vi "StandAloneTransient_Dynamic_Keithley2230_PSU_Configuration_V1.vi"(0 "VISA resource name":refnum<visa-resource-name>, 1 "POWER STATUS IN":bool, 5 "Input Array (Voltage,Current_Limit)":dbl[][](array[numeric]), 7 "Combination Scheme":u16(ring) items=["OFF", "SERIES", "PARALLEL"], 9 "Which Channels to Parallelize":u16(ring) items=["I1+I2", "ALL", "I2+I3"], 11 "error in":errorcluster) -> (3 "POWER STATUS OUT":bool, 4 "Array 4":dbl[][](array[numeric]), 6 "Array":string[](array[string]), 8 "read buffer":string, 15 "error out":errorcluster)   [LabVIEW 2019]
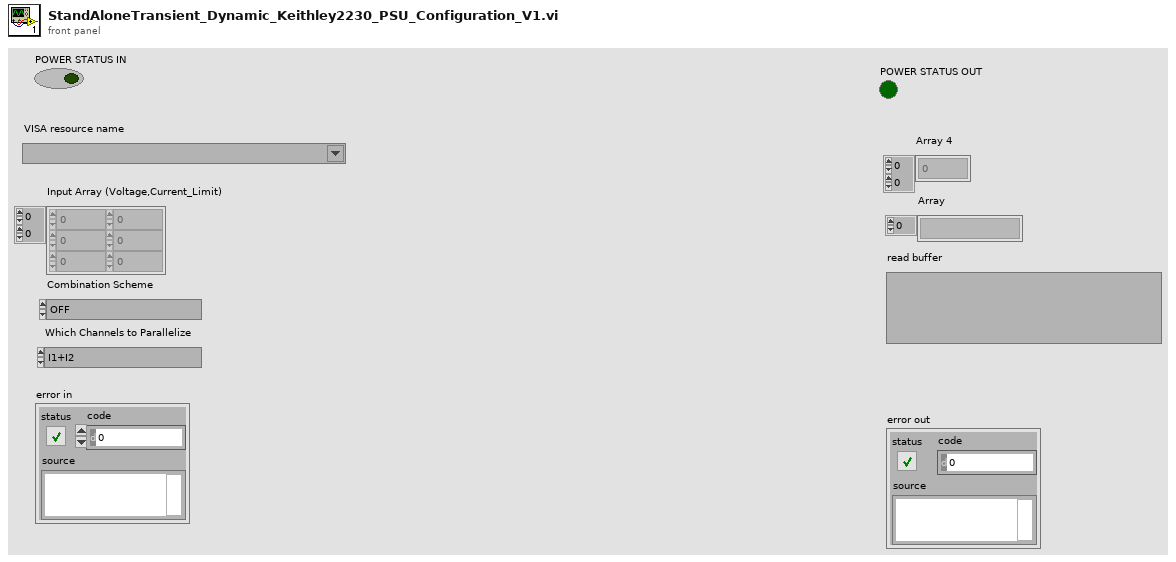
[diagram p1: front panel]
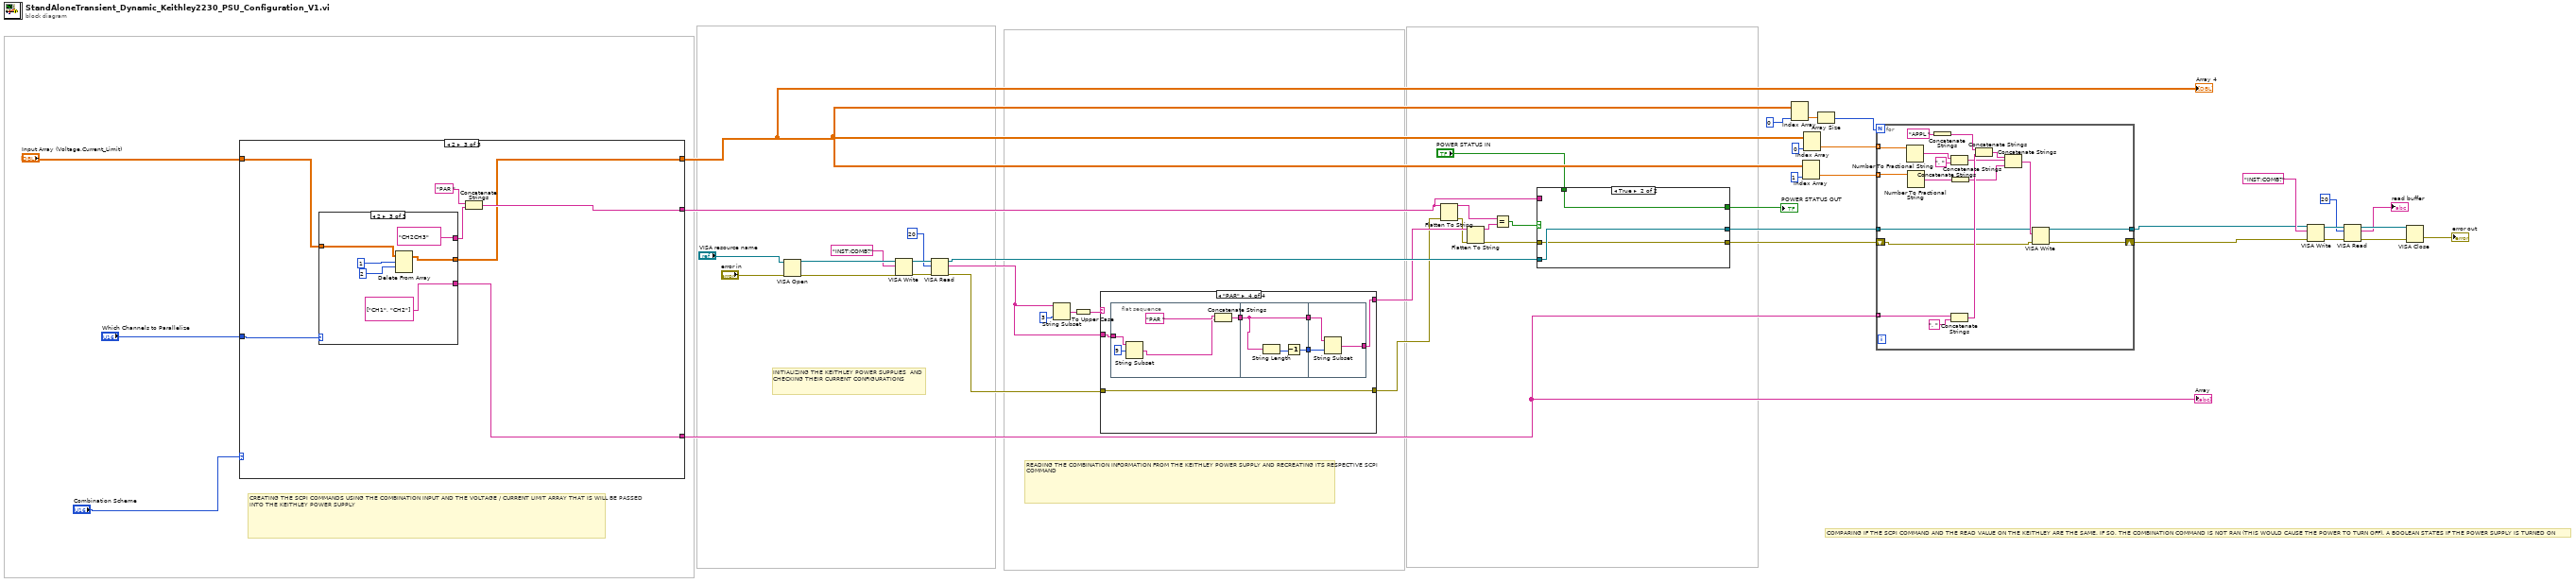
[diagram p0: block diagram]
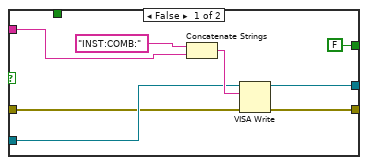
[diagram p2: hidden frame]
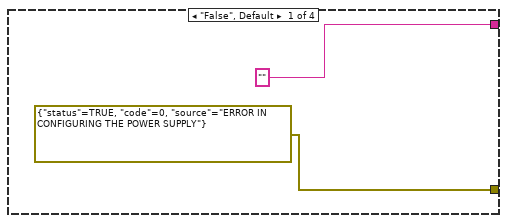
[diagram p3: hidden frame]
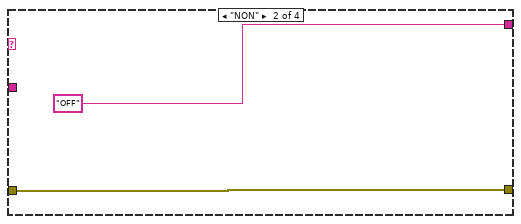
[diagram p4: hidden frame]
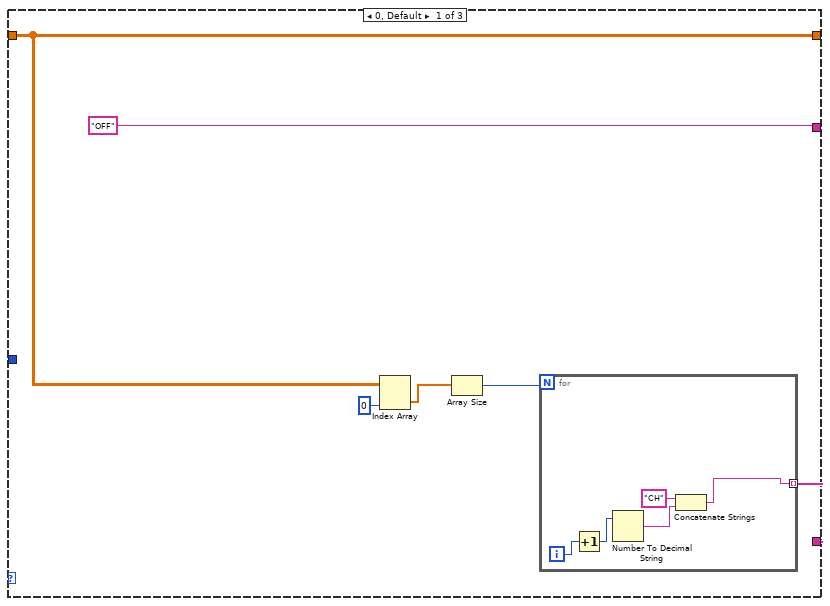
[diagram p6: hidden frame]
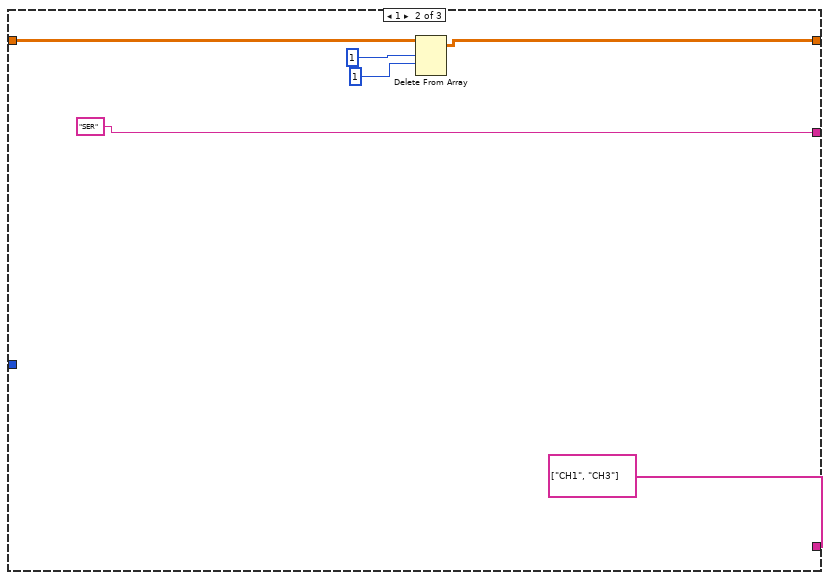
[diagram p7: hidden frame]
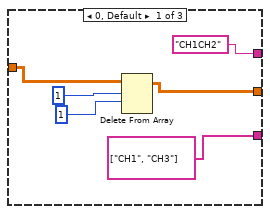
[diagram p8: hidden frame]
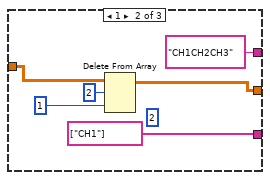
[diagram p9: hidden frame]
diagram:
  # "COMPARING IF THE SCPI COMMAND AND THE READ VALUE ON THE KEITHLEY ARE THE SAME. IF SO, THE COMBINATION COMMAND IS NOT RAN (THIS WOULD CAUSE THE POWER TO TURN OFF). A BOOLEAN STATES IF THE POWER SUPPLY IS TURNED ON"
  # "READING THE COMBINATION INFORMATION FROM THE KEITHLEY POWER SUPPLY AND RECREATING ITS RESPECTIVE SCPI COMMAND"
  # "CREATING THE SCPI COMMANDS USING THE COMBINATION INPUT AND THE VOLTAGE / CURRENT LIMIT ARRAY THAT IS WILL BE PASSED INTO THE KEITHLEY POWER SUPPLY"
  # "INITIALIZING THE KEITHLEY POWER SUPPLIES  AND CHECKING THEIR CURRENT CONFIGURATIONS"
  n1 = case shown="2" "Combination Scheme" {
    tunnel: ["OFF" "SER" w69] -> w16
    tunnel: "Which Channels to Parallelize" -> [_ _ w72]
    tunnel: "Input Array (Voltage,Current_Limit)" -> [w53 w63 w67]
    tunnel: [w53 w60 w66] -> w34
    tunnel: [w49 string[] ["CH1", "CH3"] w68] -> w35
    frame 0, Default {
      n2 = Index Array(array=w53, index (col)=0 ("disabled index (col)")) -> (element=w52:dbl[])  [unwired: 1 in]
      n3 = Array Size(array=w52) -> (size(s)=w50:i32)
      n4 = for {
        N: w50 -> [_]
        tunnel: [w55] -> w49 mode=indexing
        i -> [w58]
        n5 = Increment(x=w58) -> (x+1=w59:i32)
        n6 = Number To Decimal String(number=w59) -> (decimal integer string=w57:string)  [unwired: 1 in]
        n7 = Concatenate Strings("CH" ("string"), w57) -> (w55:string)
      }
    }
    frame 1 {
      n8 = Delete From Array(array=w63, length=1, index (row)=1) -> (array with subset deleted=w60:dbl[][])  [unwired: 1 in, 1 out]
    }
    frame 2 {
      n9 = case shown="2" w72 {
        tunnel: ["CH1CH2" "CH1CH2CH3" "CH2CH3"] -> w70
        tunnel: [string[] ["CH1", "CH3"] string[] ["CH1"] string[] ["CH1", "CH2"]] -> w68
        tunnel: w67 -> [w74 w82 w86]
        tunnel: [w73 w79 w87] -> w66
        frame 0, Default {
          n10 = Delete From Array(array=w74, length=1, index (row)=1) -> (array with subset deleted=w73:dbl[][])  [unwired: 1 in, 1 out]
        }
        frame 1 {
          (unwired) 2 ("index (row)")
          n11 = Delete From Array(array=w82, length=2, index (row)=1) -> (array with subset deleted=w79:dbl[][])  [unwired: 1 in, 1 out]
        }
        frame 2 {
          n12 = Delete From Array(array=w86, length=1, index (row)=2) -> (array with subset deleted=w87:dbl[][])  [unwired: 1 in, 1 out]
        }
      }
      n13 = Concatenate Strings("PAR ", w70) -> (w69:string)
    }
  }
  "Array 4" <- w34
  "Array" <- w35
  n14 = VISA Open(error in (no error)="error in", VISA resource name="VISA resource name") -> (VISA resource name=w31:refnum<visa-resource-name>, error out=w30:errorcluster)  [unwired: 3 in]
  n15 = VISA Write(VISA resource name=w31, write buffer="INST:COMB?", error in (no error)=w30) -> (VISA resource name out=w29:refnum<visa-resource-name>, error out=w28:errorcluster)  [unwired: 1 out]
  n16 = VISA Read(VISA resource name=w29, byte count=u32 20, error in (no error)=w28) -> (VISA resource name out=w25:refnum<visa-resource-name>, read buffer=w14:string, error out=w13:errorcluster)  [unwired: 1 out]
  n17 = String Subset(string=w14, length (rest)=3 ("length (rest)")) -> (substring=w22:string)  [unwired: 1 in]
  n18 = To Upper Case(1:w22) -> (0:w23:string)
  n19 = case shown="\"PAR\"" w23 {
    selector: w23 -> [_ _ w95 _]
    tunnel: ["" "OFF" w95 w97] -> w21
    tunnel: w14 -> [_ _ _ w102]
    tunnel: w13 -> [_ w93 w96 w101]
    tunnel: [errorcluster {"status"=TRUE, "code"=0, "source"="ERROR IN CONFIGURING THE POWER SUPPLY"} ("error out") w93 w96 w101] -> w12
    frame "False", Default {
    }
    frame "NON" {
    }
    frame "SER" {
    }
    frame "PAR" {
      n20 = flat-sequence {
        tunnel: w102 -> [w106]
        tunnel: [w103] -> w100
        tunnel: w100 -> [w109]
        tunnel: [w109] -> w99
        tunnel: [w108] -> w98
        tunnel: w99 -> [w112]
        tunnel: w98 -> [w113]
        tunnel: [w111] -> w97
        frame #0 {
          n21 = String Subset(string=w106, offset (0)=9) -> (substring=w104:string)  [unwired: 1 in]
          n22 = Concatenate Strings("PAR ", w104) -> (w103:string)
        }
        frame #1 {
          n23 = String Length(string=w109) -> (length=w110:i32)
          n24 = Decrement(x=w110) -> (x-1=w108:i32)
        }
        frame #2 {
          n25 = String Subset(string=w112, length (rest)=w113) -> (substring=w111:string)  [unwired: 1 in]
        }
      }
    }
  }
  n26 = Flatten To String(anything=w16, error in (no error)=w12) -> (data string=w19:string, error out=w18:errorcluster)  [unwired: 2 in, 1 out]
  n27 = Flatten To String(anything=w21, error in (no error)=w18) -> (data string=w20:string, error out=w17:errorcluster)  [unwired: 2 in, 1 out]
  n28 = Equal?(x=w19, y=w20) -> (x = y?=w15:bool)
  n29 = case shown="True" w15 {
    tunnel: [w119 w124] -> w38
    tunnel: [w118 w123] -> w37
    tunnel: w25 -> [w117 w124]
    tunnel: w17 -> [w116 w123]
    tunnel: w16 -> [w115 _]
    tunnel: "POWER STATUS IN" -> [_ w122]
    tunnel: [FALSE ("POWER STATUS") w122] -> w1
    frame False {
      n30 = Concatenate Strings("INST:COMB:" ("string"), w115) -> (w121:string)
      n31 = VISA Write(VISA resource name=w117, write buffer=w121, error in (no error)=w116) -> (VISA resource name out=w119:refnum<visa-resource-name>, error out=w118:errorcluster)  [unwired: 1 out]
    }
    frame True {
    }
  }
  "POWER STATUS OUT" <- w1
  n32 = Index Array(array=w34, index (col)=0 ("disabled index (col)")) -> (element=w46:dbl[])  [unwired: 1 in]
  n33 = Index Array(array=w34, index (col)=1 ("disabled index (col)")) -> (element=w41:dbl[])  [unwired: 1 in]
  n34 = Index Array(array=w34, index (col)=0 ("disabled index (col)")) -> (element=w42:dbl[])  [unwired: 1 in]
  n35 = Array Size(array=w46) -> (size(s)=w45:i32)
  n36 = for {
    N: w45 -> [_]
    tunnel: w38 -> [w127]
    tunnel: w42 -> [w137] mode=indexing
    tunnel: w41 -> [w136] mode=indexing
    tunnel: [w142] -> w4
    shift-right: [w141] -> w3
    shift-left: w37 -> [w126]
    tunnel: w35 -> [w125] mode=indexing
    n37 = Number To Fractional String(number=w137) -> (F-format string=w135:string)  [unwired: 3 in]
    n38 = Number To Fractional String(number=w136) -> (F-format string=w133:string)  [unwired: 3 in]
    n39 = Concatenate Strings("APPL " ("string")) -> (w138:string)
    n40 = Concatenate Strings(w135, ", " ("string")) -> (w131:string)
    n41 = Concatenate Strings(w125, ", " ("string")) -> (w139:string)
    n42 = Concatenate Strings(w133) -> (w130:string)
    n43 = Concatenate Strings(w138, w139) -> (w132:string)
    n44 = Concatenate Strings(w132, w131, w130) -> (w129:string)
    n45 = VISA Write(VISA resource name=w127, write buffer=w129, error in (no error)=w126) -> (VISA resource name out=w142:refnum<visa-resource-name>, error out=w141:errorcluster)  [unwired: 1 out]
  }
  n46 = VISA Write(VISA resource name=w4, write buffer="INST:COMB?", error in (no error)=w3) -> (VISA resource name out=w11:refnum<visa-resource-name>, error out=w10:errorcluster)  [unwired: 1 out]
  n47 = VISA Read(VISA resource name=w11, byte count=u32 20, error in (no error)=w10) -> (VISA resource name out=w7:refnum<visa-resource-name>, read buffer=→"read buffer":string, error out=w6:errorcluster)  [unwired: 1 out]
  n48 = VISA Close(VISA resource name=w7, error in (no error)=w6) -> (error out=→"error out":errorcluster)
